vi "Writes_fkcommand.vi"(8 "error in (no error)":errorcluster, 10 "fkcommand":T1 {"执行结果定义" items=["执行成功"=1, "执行失败，但不知道原因"=2, "命令请求条件错误"=3, "通讯超时"=4, "系统繁忙不能执行"=5, "系统故障"=6, "没有数据"=100]}, 11 "object in":refnum<class "212format_work.lvclass">) -> (0 "error out":errorcluster, 3 "object out":refnum<class "212format_work.lvclass">)   [LabVIEW 2016, in "212format_work.lvclass"]
uses:
  212format_work.lvclass
  212format_work.lvclass/212format_work.ctl
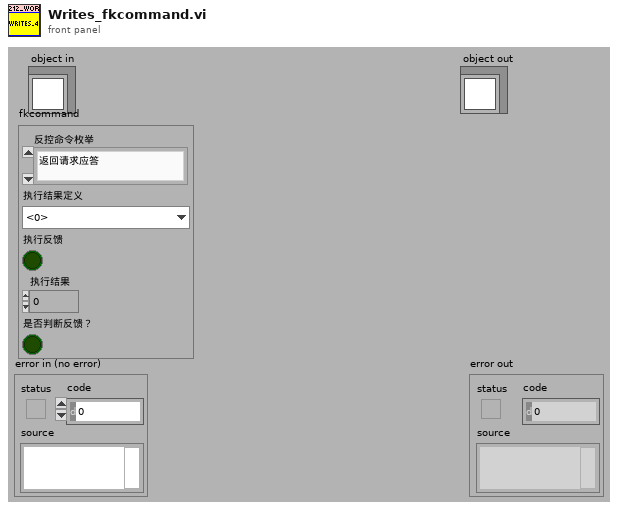
[diagram p1: front panel]
types:
  T1 = typedef "212format_work.lvclass/fkcommand控件.ctl" = cluster{"反控命令枚举":enum16{"返回请求应答", "返回执行结果"}, "执行结果定义":u16, "执行反馈":bool, "执行结果":u16, "是否判断反馈？":bool}
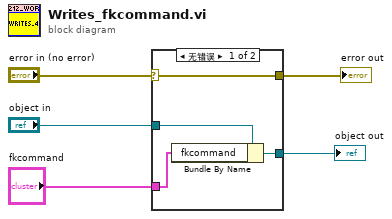
[diagram p0: block diagram]
diagram:
  n1 = case shown="无错误" "error in (no error)" {
    selector: "error in (no error)" -> [w9 w11]
    tunnel: [w9 w11] -> w4
    tunnel: [w7 w10] -> w2
    tunnel: "object in" -> [w8 w10]
    tunnel: "fkcommand" -> [w6 _]
    frame No Error {
      n2 = Bundle By Name(cluster=w8, "fkcommand"=w6) -> (w7:refnum<class "212format_work.lvclass">)
    }
    frame Error {
    }
  }
  "error out" <- w4
  "object out" <- w2
